vi "Get Supported SG Path Class Names.vi"(0 "SG Path PM Accessor in":refnum<class "SG 2250 Path Accessor.lvclass">, 11 "error in (no error)":errorcluster) -> (4 "SG Path PM Accessor out":refnum<class "SG 2250 Path Accessor.lvclass">, 6 "Supported SG Path Class Names":string[](array[string]), 15 "error out":errorcluster)   [LabVIEW 2023, in "NI-568x RF Power Meter.lvlib" / "SG 2250 Path Accessor.lvclass"]
uses:
  SG 2250 Path Accessor.lvclass
  RFPM/Scalar/Paths/SG SC2250 Path/SG SC2250 Path.lvclass
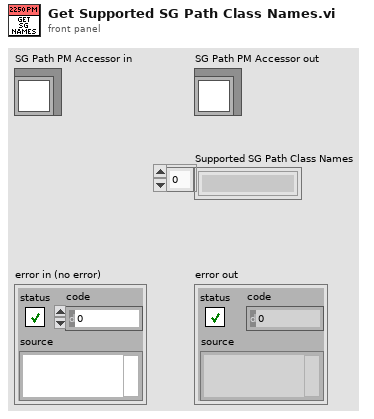
[diagram p1: front panel]
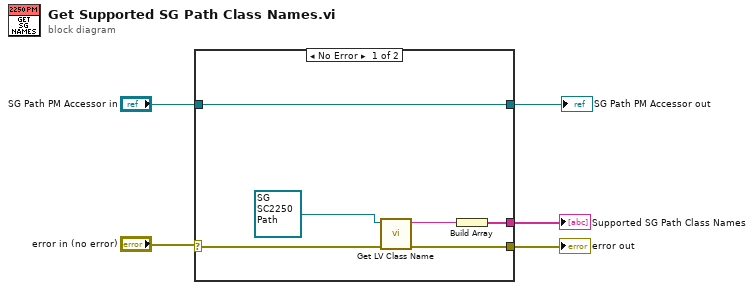
[diagram p0: block diagram]
diagram:
  n1 = case shown="No Error" "error in (no error)" {
    selector: "error in (no error)" -> [w9 w13]
    tunnel: [w8 w13] -> w2
    tunnel: [w11 w12] -> w3
    tunnel: "SG Path PM Accessor in" -> [w11 w12]
    tunnel: [w10 _] -> w1
    frame No Error {
      n2 = call <vilib>:"Get LV Class Name.vi"("error in (no error)"=w9, "object"=refnum<class "SG SC2250 Path.lvclass"> refnum ("RFFixtureCharact.Scalar.lvlib:SG SC2250 Path.lvclass")) -> ("error out"=w8:errorcluster, "class name"=w6:string)  [unwired: 8 in]
      n3 = Build Array(w6) -> (w10:string[])
    }
    frame Error {
    }
  }
  "error out" <- w2
  "SG Path PM Accessor out" <- w3
  "Supported SG Path Class Names" <- w1
